vi "Update QV-Status on ACFP.vi"(8 "Error In":errorcluster, 11 "KIT-QVA in":refnum<class "KIT-QVA.lvclass">) -> (0 "Error Out":errorcluster, 3 "KIT-QVA out":refnum<class "KIT-QVA.lvclass">)   [LabVIEW 2014, in "KIT-QVA.lvlib" / "KIT-QVA.lvclass"]
doc: "Update KIT-QV status on FP of Acotre Core.vi."
uses:
  KIT-QVA.lvclass
  KIT-QVA.lvclass/KIT-QVA.ctl
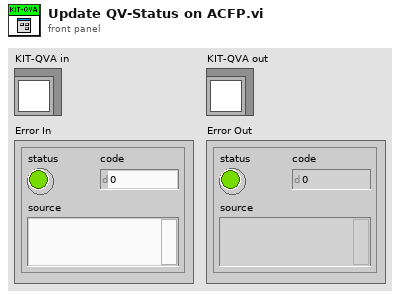
[diagram p1: front panel]
types:
  T1 = cluster{"System Test":bool, "Test Mode":bool, "Fault":bool, "Quench":bool, "U/T Fault":bool, "Bus Error":bool, "System Fault":bool, "Control Mode":bool}
  T2 = cluster{"System Test":bool, "Test Mode":bool, "Fault":bool, "Quench":bool, "U/T Fault":bool, "Bus Error":bool, "System Fault":bool, "Reserved":bool}[]
  T3 = cluster{"Q1+":bool, "Q1-":bool, "Q2+":bool, "Q2-":bool, "Mute":bool, "STest-Bit":bool, "QD1":bool, "QD2":bool}[]
  T4 = cluster{"Detector Status":cluster{"System Test":bool, "Test Mode":bool, "Fault":bool, "Quench":bool, "U/T Fault":bool, "Bus Error":bool, "System Fault":bool, "Reserved":bool}, "Hardware Status":cluster{"Q1+":bool, "Q1-":bool, "Q2+":bool, "Q2-":bool, "Mute":bool, "STest-Bit":bool, "QD1":bool, "QD2":bool}, "ADC Raw":i16, "Volatage":dbl[unit]}
  T5 = cluster{"Detector Update":timestamp, "Temperature":dbl[unit], cluster{"Detector Status":cluster{"System Test":bool, "Test Mode":bool, "Fault":bool, "Quench":bool, "U/T Fault":bool, "Bus Error":bool, "System Fault":bool, "Reserved":bool}, "Hardware Status":cluster{"Q1+":bool, "Q1-":bool, "Q2+":bool, "Q2-":bool, "Mute":bool, "STest-Bit":bool, "QD1":bool, "QD2":bool}, "ADC Raw":i16, "Volatage":dbl[unit]}[]}
  T6 = cluster{"Rack Update":timestamp, "Rack Status":cluster{"System Test":bool, "Test Mode":bool, "Fault":bool, "Quench":bool, "U/T Fault":bool, "Bus Error":bool, "System Fault":bool, "Control Mode":bool}, cluster{"Detector Update":timestamp, "Temperature":dbl[unit], cluster{"Detector Status":cluster{"System Test":bool, "Test Mode":bool, "Fault":bool, "Quench":bool, "U/T Fault":bool, "Bus Error":bool, "System Fault":bool, "Reserved":bool}, "Hardware Status":cluster{"Q1+":bool, "Q1-":bool, "Q2+":bool, "Q2-":bool, "Mute":bool, "STest-Bit":bool, "QD1":bool, "QD2":bool}, "ADC Raw":i16, "Volatage":dbl[unit]}[]}}
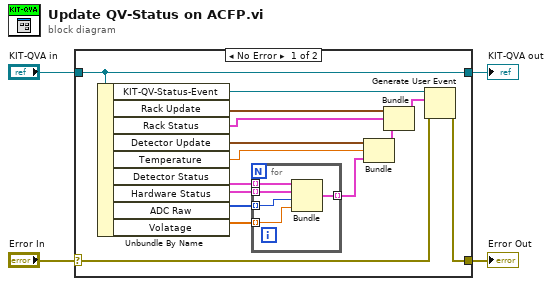
[diagram p0: block diagram]
diagram:
  n1 = case shown="No Error" "Error In" {
    selector: "Error In" -> [w17 w26]
    tunnel: [w16 w26] -> w3
    tunnel: [w19 w25] -> w1
    tunnel: "KIT-QVA in" -> [w19 w25]
    frame No Error {
      n2 = Unbundle By Name(w19) -> ("KIT-QV-Status-Event"=w18:refnum<user-event>, "Rack Update"=w15:timestamp, "Rack Status"=w14:T1, "Detector Update"=w13:timestamp, "Temperature"=w5:dbl[unit], "Detector Status"=w10:T2, "Hardware Status"=w9:T3, "ADC Raw"=w8:i16[], "Volatage"=w7:dbl[unit][])
      n3 = for {
        tunnel: w10 -> [w24] mode=indexing
        tunnel: w9 -> [w23] mode=indexing
        tunnel: w8 -> [w22] mode=indexing
        tunnel: w7 -> [w21] mode=indexing
        tunnel: [w20] -> w6 mode=indexing
        n4 = Bundle("Detector Status"=w24, "Hardware Status"=w23, "ADC Raw"=w22, "Volatage"=w21) -> (w20:T4)  [unwired: 1 in]
      }
      n5 = Bundle("Detector Update"=w13, "Temperature"=w5, w6) -> (w12:T5)  [unwired: 1 in]
      n6 = Bundle("Rack Update"=w15, "Rack Status"=w14, w12) -> (w11:T6)  [unwired: 1 in]
      n7 = Generate User Event(user event=w18, event data cluster=w11, error in=w17) -> (error out=w16:errorcluster)  [unwired: 1 in, 1 out]
    }
    frame Error {
    }
  }
  "Error Out" <- w3
  "KIT-QVA out" <- w1
